vi "Open File Do.vi"(8 "error in (no error)":errorcluster, 10 "New File Path":path, 11 "File Writer in":refnum<class "File Writer.lvclass">) -> (0 "error out":errorcluster, 1 "Success?":bool, 3 "File Writer out":refnum<class "File Writer.lvclass">)   [LabVIEW 2020, in "File Writer.lvlib" / "File Writer.lvclass"]
doc: "Open a file.\nDefault implementation prevents saving of data. Do not call the parent method to the top level."
uses:
  File Writer.lvclass
  File Writer.lvclass/File Writer.ctl
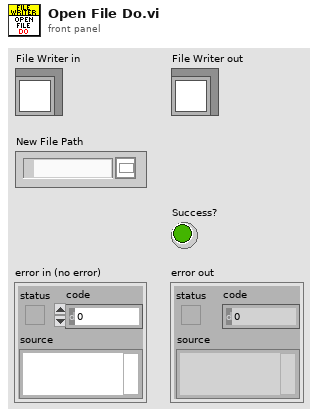
[diagram p1: front panel]
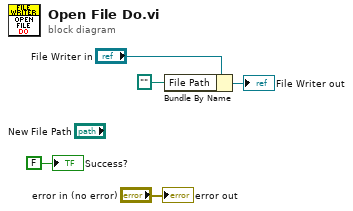
[diagram p0: block diagram]
diagram:
  n1 = Bundle By Name(cluster="File Writer in", "File Path"=path "") -> (→"File Writer out":refnum<class "File Writer.lvclass">)
  "error out" <- "error in (no error)"
  "Success?" <- FALSE ("Success?")
